vi "Initialise.vi"(8 "error in (no error)":errorcluster, 10 "Instrument Ref":string, 11 "Keysight 5700C in":refnum<class "Keysight 5700C.lvclass">) -> (0 "error out":errorcluster, 3 "Keysight 5700C out":refnum<class "Keysight 5700C.lvclass">)   [LabVIEW 2019, in "Concrete.lvlib" / "Keysight 5700C.lvclass"]
uses:
  Keysight 5700C.lvclass
  Keysight 5700C.lvclass/Keysight 5700C.ctl
  Harware Abstraction/Analog out/Analog out.lvclass
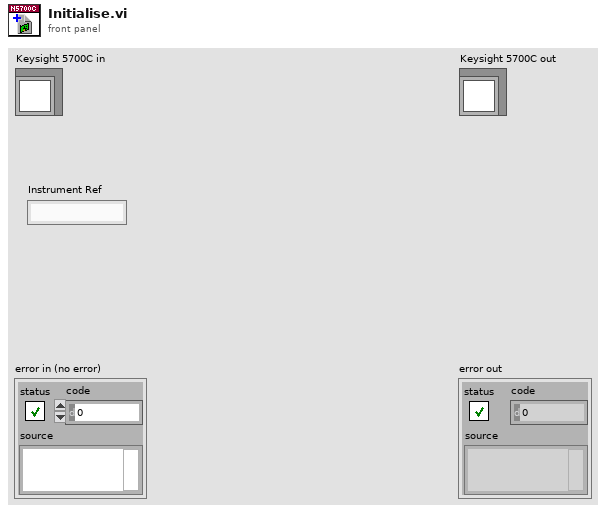
[diagram p1: front panel]
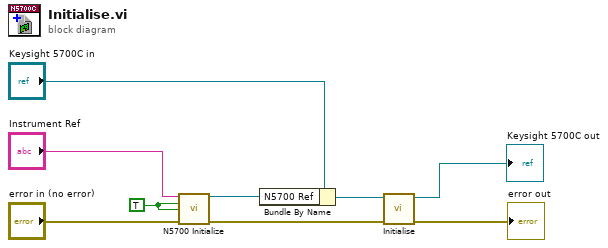
[diagram p0: block diagram]
diagram:
  w2 = TRUE ("id query (Yes)")
  n1 = call <instrlib>:"N5700 Initialize.vi"("VISA name"="Instrument Ref", "ID Query (T)"=w2, "Reset (T)"=w2, "error in (no error)"="error in (no error)") -> ("VISA out"=w1:refnum<visa-resource-name>, "error out"=w4:errorcluster)  [unwired: 10 in]
  n2 = Bundle By Name(cluster="Keysight 5700C in", "N5700 Ref"=w1) -> (w6:refnum<class "Keysight 5700C.lvclass">)
  n3 = call-parent "Initialise.vi"("error in (no error)"=w4, "Instrument in"=w6) -> ("error out"=→"error out":errorcluster, "Instrument out"=→"Keysight 5700C out":refnum<class "Keysight 5700C.lvclass">)  [unwired: 8 in]
